vi "vision system.vi"() -> ()   [LabVIEW 2018]
uses:
  <vilib>/userdefined/High Color/IMAQdx.ctl
  <vilib>/vision/Measure.llb/Straight Edge Options.ctl
  <vilib>/vision/Measure.llb/Straight Edge Process.ctl
  <vilib>/vision/Measure.llb/Edge Options.ctl
  <vilib>/vision/Measure.llb/Edge Polarity.ctl
  <vilib>/Utility/file.llb/Read Delimited Spreadsheet (string).vi
  <vilib>/Utility/file.llb/Read Delimited Spreadsheet (DBL).vi
  <vilib>/Utility/file.llb/Write Delimited Spreadsheet (DBL).vi
  <vilib>/vision/driver/NI_Vision_Acquisition_Software.lvlib
  <vilib>/vision/NI_Vision_Development_Module.lvlib
panel:
  out "Jednostka ostatnia":string
  out "Ostatnia zapisana wartość:":dbl
  in  "Zmiana zakresu":i32 min=0
  out "Miernik":string
  in  "Zmiana mierzonej wielkości":i32 min=0
  out "Zakresy w kolumnach":dbl[][](array[numeric])
  out "Naglowki":string[][](array[string])
  in  "Plik z zakresami":path=path "C:/Users/Darek/Desktop/mierniki_zakresy.csv"
  in  "Skoroszyt csv do zapisu pomiarów":path=path "C:/Users/Darek/Desktop/wyniki_pomiarow.csv"
  in  "Zapis":bool
  out "Mnożnik zakresu":dbl
  in  "Kierunek ruchu wskazówki":T1(ring)
  out "Jednostka kopia":string
  out "Kąt wskazówki":dbl
  in  "Tryb zoptymalizowany":bool=TRUE
  in  "Opcje linii wskazówki":T2={"Edge Polarity"=0, "Kernel Size"=3, "Width"=3, "Minimum Edge Strength"=10.0, "Interpolation Type"=enum."Bilinear Fixed", "Data Processing Method"=enum."Average"} {"Edge Polarity" items=["All Edges", "Rising Edges", "Falling Edges"]; "Minimum Edge Strength" format="%.2f"; "Width" step=2; "Kernel Size" step=2}
  in  "Kierunek szukania":u32(ring) items=["Left to Right", "Right to Left", "Top to Bottom", "Bottom to Top"]
  in  "Dopasownie linii wskazówki":T4={"Number of Lines"=1, "Type"=enum."Best Edge Rake", "Min. Score"=10.0, "Max. Score"=1000.0, "Orientation"=0.0, "Angle Range"=10.0, "Angle Tolerance"=1.0, "Step Size"=3, "Min. SNR (db)"=0.0, "Min. Points (%)"=25.0, "Hough Iterations"=5} {"Min. Points (%)" min=0.0 max=100.0; "Min. SNR (db)" min=0.0; "Max. Score" min=0.0 max=1024.0; "Min. Score" min=0.0 max=1024.0 step=1.0}
  out "Kąt prawej linii":dbl
  out "Kąt lewej linii":dbl
  out "WYNIK":dbl
  out "Jednostka":string
  out "Zakres":dbl
  in  "Rodzaj skali":enum16{"Skale liniowe", "Ohmy V640"}(ring)
  in  "Znajdowanie \nwskazówki":bool
  out "Boolean 3":bool
  out "Kąt wskazówki raw":dbl
  out "Rozstaw podziałki\n w stopniach":dbl
  out "Kąt prawej linii raw":dbl
  out "Kąt lewej linii raw":dbl
  in  "Opcje prawej linii":T6={"Search Direction"=1, "Edge Options"={"Edge Polarity"=1, "Kernel Size"=3, "Width"=3, "Minimum Edge Strength"=10.0, "Interpolation Type"=enum."Bilinear Fixed", "Data Processing Method"=enum."Average"}, "Show Search Area"=FALSE, "Show Search Lines"=FALSE, "Show Edges Found"=FALSE, "Show Result"=FALSE, "Search Area Color"=65280, "Search Lines Color"=255, "Edge Locations Color"=16776960, "Result Color"=16711680, "Overlay Group Name"=""} {"Edge Options"."Edge Polarity" items=["All Edges", "Rising Edges", "Falling Edges"]; "Edge Options"."Minimum Edge Strength" format="%.2f"; "Edge Options"."Width" step=2; "Edge Options"."Kernel Size" step=2; "Search Direction" items=["Left to Right", "Right to Left", "Top to Bottom", "Bottom to Top"]}
  in  "Opcje lewej linii":T6={"Search Direction"=0, "Edge Options"={"Edge Polarity"=1, "Kernel Size"=3, "Width"=3, "Minimum Edge Strength"=10.0, "Interpolation Type"=enum."Bilinear Fixed", "Data Processing Method"=enum."Average"}, "Show Search Area"=FALSE, "Show Search Lines"=FALSE, "Show Edges Found"=FALSE, "Show Result"=FALSE, "Search Area Color"=65280, "Search Lines Color"=255, "Edge Locations Color"=16776960, "Result Color"=16711680, "Overlay Group Name"=""} {"Edge Options"."Edge Polarity" items=["All Edges", "Rising Edges", "Falling Edges"]; "Edge Options"."Minimum Edge Strength" format="%.2f"; "Edge Options"."Width" step=2; "Edge Options"."Kernel Size" step=2; "Search Direction" items=["Left to Right", "Right to Left", "Top to Bottom", "Bottom to Top"]}
  in  "Dop. prawej linii":T4={"Number of Lines"=1, "Type"=enum."First Edge Rake", "Min. Score"=10.0, "Max. Score"=1000.0, "Orientation"=0.0, "Angle Range"=45.0, "Angle Tolerance"=1.0, "Step Size"=7, "Min. SNR (db)"=0.0, "Min. Points (%)"=25.0, "Hough Iterations"=5} {"Min. Points (%)" min=0.0 max=100.0; "Min. SNR (db)" min=0.0; "Max. Score" min=0.0 max=1024.0; "Min. Score" min=0.0 max=1024.0 step=1.0}
  out "Boolean 2":bool
  in  "Znajdowanie \nprostych":bool
  out "Boolean":bool
  in  "Dopasowanie \nwzorca":bool
  in  "Dop. lewej linii":T4={"Number of Lines"=1, "Type"=enum."First Edge Rake", "Min. Score"=10.0, "Max. Score"=1000.0, "Orientation"=0.0, "Angle Range"=45.0, "Angle Tolerance"=1.0, "Step Size"=7, "Min. SNR (db)"=0.0, "Min. Points (%)"=25.0, "Hough Iterations"=5} {"Min. Points (%)" min=0.0 max=100.0; "Min. SNR (db)" min=0.0; "Max. Score" min=0.0 max=1024.0; "Min. Score" min=0.0 max=1024.0 step=1.0}
  out "Podglad":T7(plugin-control)
  out "Miernik wykryty":bool
  in  "stop":bool
  out "Błąd pracy systemu":errorcluster
  out "Wzorzec":T7(plugin-control)
  in  "Paramtery\ndopasowania":T8={"Number of Matches Requested"=1, "Minimum Match Score"=800.0, "Angle Ranges"=[]}
  in  "Sciezka \nobrazu wzorcowego":path=path "C:/Users/Darek/Desktop/templates/V640_temp_8bit.png"
  out "Błąd akwizycji obrazu":errorcluster
  in  "Kamera":T9="cam1"
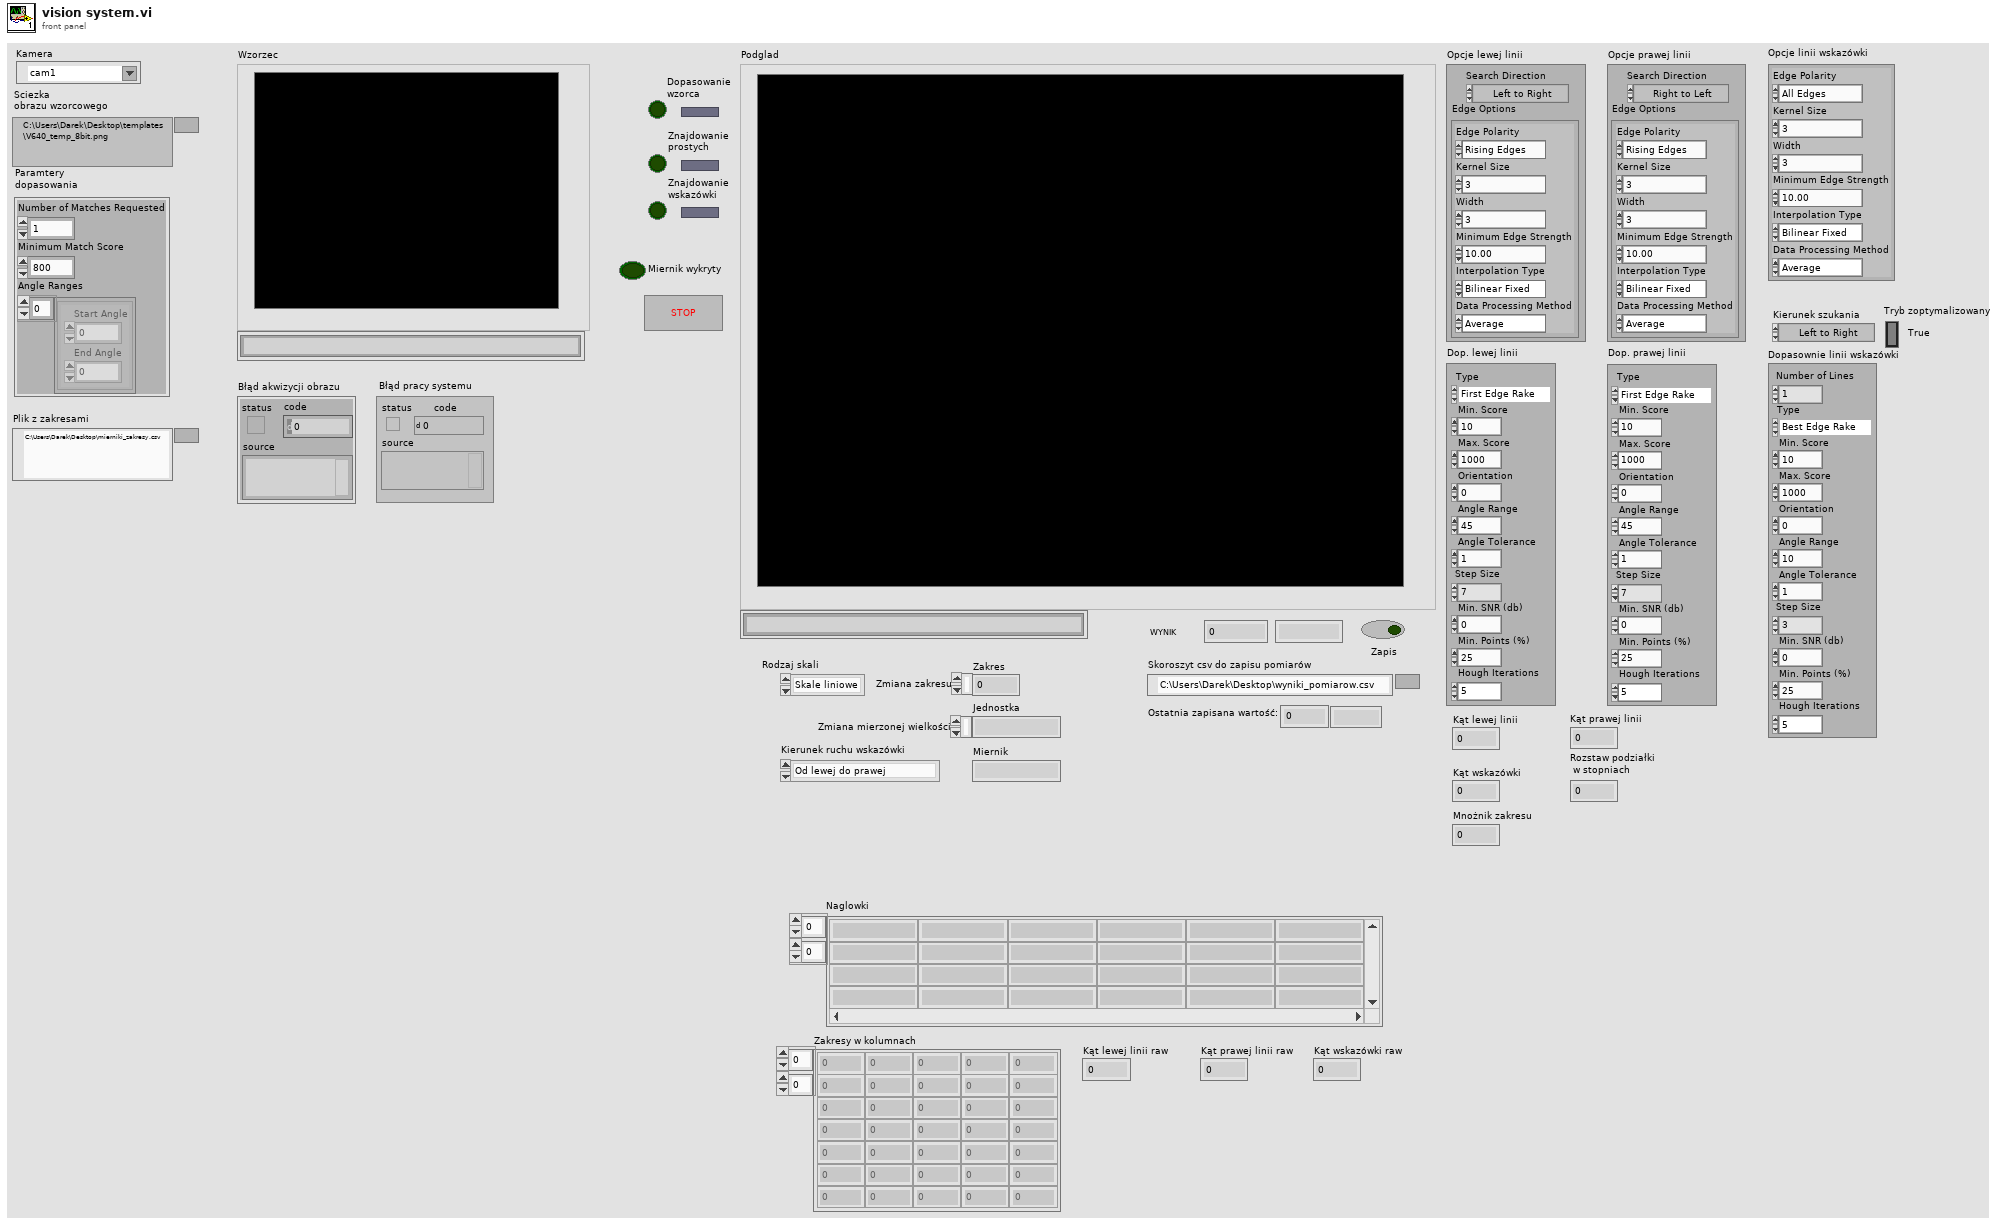
[diagram p1: front panel]
types:
  T1 = enum16{"Od lewej do prawej", "Od prawej do lewej"}
  T2 = typedef "Edge Options.ctl" = cluster{"Edge Polarity":T3, "Kernel Size":u32, "Width":u32, "Minimum Edge Strength":sgl, "Interpolation Type":enum32{"Zero Order", "Bilinear", "Quadratic", "Cubic", "Bilinear Fixed"}, "Data Processing Method":enum32{"Average", "Median"}}
  T3 = typedef "Edge Polarity.ctl" = u32
  T4 = typedef "Straight Edge Options.ctl" = cluster{"Number of Lines":i32, "Type":T5, "Min. Score":dbl, "Max. Score":dbl, "Orientation":dbl, "Angle Range":dbl, "Angle Tolerance":dbl, "Step Size":u32, "Min. SNR (db)":dbl, "Min. Points (%)":dbl, "Hough Iterations":i32}
  T5 = typedef "Straight Edge Process.ctl" = enum32{"First Edge Rake", "Best Edge Rake", "Hough Edge Rake", "First Edge Projection", "Best Edge Projection"}
  T6 = cluster{"Search Direction":u32, "Edge Options":T2, "Show Search Area":bool, "Show Search Lines":bool, "Show Edges Found":bool, "Show Result":bool, "Search Area Color":u32, "Search Lines Color":u32, "Edge Locations Color":u32, "Result Color":u32, "Overlay Group Name":string}
  T7 = typedef "IMAQ Image.ctl" = refnum<image>
  T8 = cluster{"Number of Matches Requested":i32, "Minimum Match Score":sgl, "Angle Ranges":cluster{"Start Angle":sgl, "End Angle":sgl}[]}
  T9 = typedef "IMAQdx.ctl" = refnum<k21>
  T10 = typedef "Image Type" = u32
  T11 = cluster{i32, "Y Resolution":i32, "X Resolution":i32, i32, dbl}
  T12 = typedef "ROI Descriptor" = cluster{"Global Rectangle":i32[], "Contours":cluster{"ID":enum32{"External", "Internal"}, "Type":u32, "Coordinates":i32[]}[]}
  T13 = cluster{"Position":cluster{"x":sgl, "y":sgl}, "Angle":sgl, "Scale":sgl, "Score":sgl, "Bounding Box":cluster{"x":sgl, "y":sgl}[]}[]
  T14 = typedef "IMAQ Coordinate System" = cluster{"Reference System":cluster{"Origin":cluster{"X":sgl, "Y":sgl}, "Angle (deg)":sgl, "Axis Reference":u32}, "Measurement System":cluster{"Origin":cluster{"X":sgl, "Y":sgl}, "Angle (deg)":sgl, "Axis Reference":u32}}
  T15 = cluster{"Point1 (Pixels)":cluster{"X":sgl, "Y":sgl}, "Point2 (Pixels)":cluster{"X":sgl, "Y":sgl}, "Point1 (Real-World)":cluster{"X":sgl, "Y":sgl}, "Point2 (Real-World)":cluster{"X":sgl, "Y":sgl}, "Angle (Pixel)":dbl, "Angle (Real-World)":dbl, "Score":dbl, "Straightness":dbl, "Average SNR (db)":dbl, "Calibration Valid":bool}[]
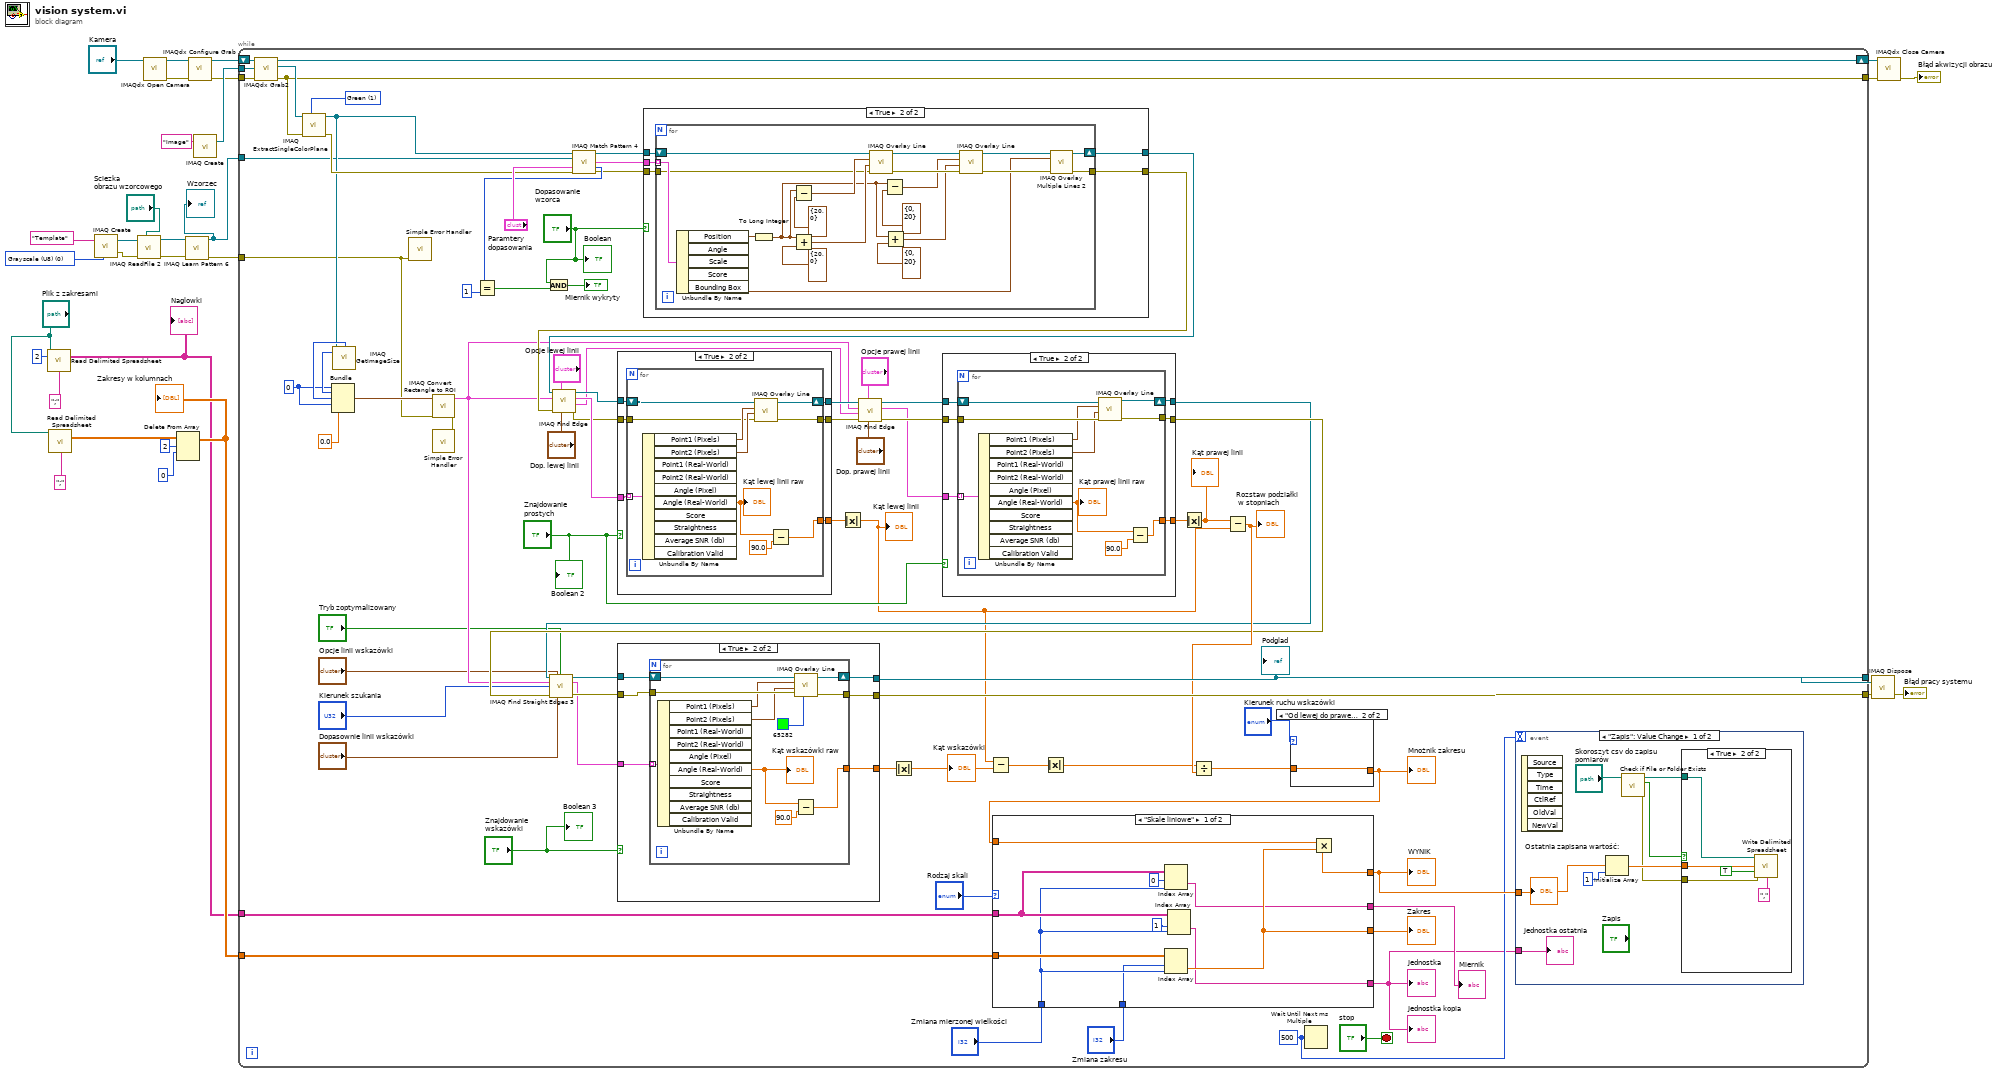
[diagram p0: block diagram]
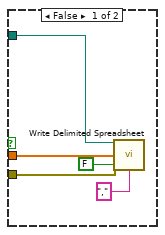
[diagram p2: hidden frame]
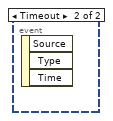
[diagram p3: hidden frame]
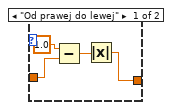
[diagram p4: hidden frame]
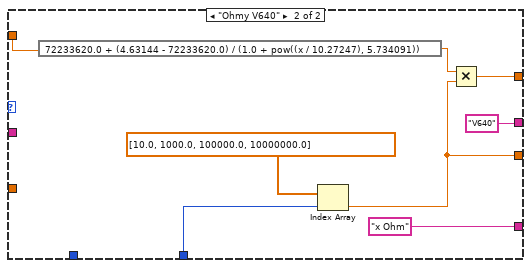
[diagram p5: hidden frame]
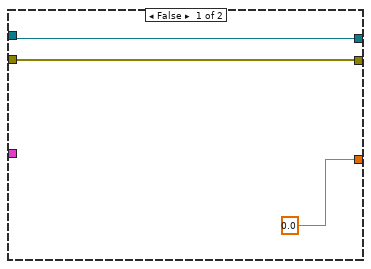
[diagram p6: hidden frame]
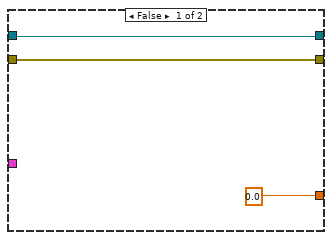
[diagram p7: hidden frame]
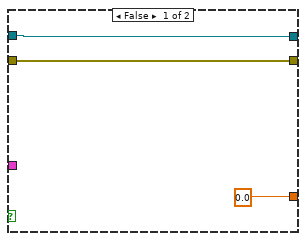
[diagram p8: hidden frame]
diagram:
  w19 = T10 0 items=["Grayscale (U8)", "Grayscale (I16)", "Grayscale (SGL)", "Complex (CSG)", "RGB (U32)", "HSL (U32)", "RGB (U64)", "Grayscale (U16)"] ("Image Type")
  n1 = call-poly <vilib>:"Read Delimited Spreadsheet.vi"("file path (dialog if empty)"="Plik z zakresami", "number of rows (all:-1)"=2, "delimiter (\\t)"=";" ("delimiter (\\t)")) -> ("all rows"=w1:string[][])  [unwired: 7 in, 5 out]
  "Naglowki" <- w1
  n2 = call-poly <vilib>:"Read Delimited Spreadsheet.vi"("file path (dialog if empty)"="Plik z zakresami", "delimiter (\\t)"=";" ("delimiter (\\t)")) -> ("all rows"=w5:dbl[][])  [unwired: 8 in, 5 out]
  n3 = call "IMAQ Create"("Image Name"="Template", "Image Type"=w19) -> ("New Image"=w15:T7, "error out"=w16:errorcluster)  [unwired: 3 in]
  n4 = call "IMAQ ReadFile 2"("File Path"="Sciezka \nobrazu wzorcowego", "error in (no error)"=w16, "Image"=w15) -> ("error out"=w14:errorcluster, "Image Out"=w12:T7)  [unwired: 4 in, 3 out]
  n5 = call <vilib>:"IMAQdx Open Camera.vi"("Session In"="Kamera") -> ("error out"=w28:errorcluster, "Session Out"=w31:T9)  [unwired: 9 in]
  n6 = Delete From Array(array=w5, length=2, index (row)=0) -> (array with subset deleted=w2:dbl[][])  [unwired: 1 in, 1 out]
  "Zakresy w kolumnach" <- w2
  n7 = call "IMAQ Learn Pattern 6"("Image"=w12, "error in (no error)"=w14) -> ("Template Image Out"=w11:T7, "error out"=w10:errorcluster)  [unwired: 11 in, 1 out]
  "Wzorzec" <- w11
  n8 = call <vilib>:"IMAQdx Configure Grab.vi"("error in"=w28, "Session In"=w31) -> ("error out"=w22:errorcluster, "Session Out"=w30:T9)  [unwired: 8 in]
  n9 = call "IMAQ Create"("Image Name"="Image") -> ("New Image"=w24:T7)  [unwired: 4 in, 1 out]
  n10 = while {
    shift-right: [w108] -> w27
    shift-left: w30 -> [w109]
    tunnel: w24 -> [w105]
    tunnel: w22 -> [w101]
    tunnel: [w100] -> w21
    tunnel: [w70] -> w18
    tunnel: [w67] -> w17
    tunnel: w11 -> [w39]
    tunnel: w10 -> [w38]
    tunnel: w2 -> [w37]
    tunnel: w1 -> [w36]
    stop <- "stop" stop-if-true
    w40 = u32 500 ("millisecond multiple")
    w89 = 0
    w106 = 1 items=["Red", "Green", "Blue", "Hue", "Saturation", "Luminance", "Value", "Intensity"] ("Color Plane")
    n11 = call <vilib>:"IMAQdx Grab2.vi"("error in"=w101, "Image In"=w105, "Session In"=w109) -> ("error out"=w100:errorcluster, "Image Out"=w107:T7, "Session Out"=w108:T9)  [unwired: 5 in, 1 out]
    n12 = call "IMAQ ExtractSingleColorPlane"("Color Plane"=w106, "error in (no error)"=w100, "Image Src"=w107) -> ("error out"=w94:errorcluster, "Image Dst Out"=w86:T7)  [unwired: 7 in]
    n13 = call "IMAQ GetImageSize"("Image"=w86) -> ("Y Resolution"=w91:i32, "X Resolution"=w90:i32)  [unwired: 3 in, 1 out]
    n14 = Bundle(w89, "Y Resolution"=w91, "X Resolution"=w90, w89, 0.0) -> (w87:T11)  [unwired: 1 in]
    n15 = call <vilib>:"Simple Error Handler.vi"("error in (no error)"=w38) -> ()  [unwired: 4 in, 5 out]
    n16 = call "IMAQ Convert Rectangle to ROI"("error in (no error)"=w38, "Rectangle"=w87) -> ("error out"=w92:errorcluster, "ROI Descriptor"=w54:T12)  [unwired: 7 in]
    n17 = call <vilib>:"Simple Error Handler.vi"("error in (no error)"=w92) -> ()  [unwired: 4 in, 5 out]
    n18 = call "IMAQ Match Pattern 4"("Image"=w86, "Template Image"=w39, "Parameters"="Paramtery\ndopasowania", "error in (no error)"=w94) -> ("Image (duplicate)"=w64:T7, "Matches (pixel)"=w63:T13, "Number of Matches"=w62:i32, "error out"=w61:errorcluster)  [unwired: 7 in, 1 out]
    n19 = Equal?(x=w62, y=1) -> (x = y?=w85:bool)
    n20 = And(x="Dopasowanie \nwzorca", y=w85) -> (x .and. y?=→"Miernik wykryty":bool)
    n21 = case shown="True" "Dopasowanie \nwzorca" {
      tunnel: w64 -> [w211 w216]
      tunnel: w61 -> [w210 w215]
      tunnel: w63 -> [_ w214]
      tunnel: [w211 w213] -> w95
      tunnel: [w210 w212] -> w93
      frame False {
      }
      frame True {
        n22 = for {
          shift-right: [w217] -> w213
          shift-left: w216 -> [w221]
          tunnel: w214 -> [w232] mode=indexing
          tunnel: w215 -> [w220]
          tunnel: [w219] -> w212
          n23 = Unbundle By Name(w232) -> ("Position"=w231:cluster{"x":sgl, "y":sgl}, "Bounding Box"=w218:cluster{"x":sgl, "y":sgl}[])  [unwired: 3 out]
          n24 = To Long Integer(number=w231) -> (32bit integer=w225:cluster{"x":i32, "y":i32})
          n25 = Subtract(x=w225, y=cluster{"x":i32, "y":i32} {"x"=20, "y"=0}) -> (x-y=w228:cluster{"x":i32, "y":i32})
          n26 = Add(x=w225, y=cluster{"x":i32, "y":i32} {"x"=20, "y"=0}) -> (x+y=w227:cluster{"x":i32, "y":i32})
          n27 = call "IMAQ Overlay Line"("error in (no error)"=w220, "End Point"=w227, "Start Point"=w228, "Image"=w221) -> ("error out"=w234:errorcluster, "Image Out"=w235:T7)  [unwired: 6 in]
          n28 = Subtract(x=w225, y=cluster{"x":i32, "y":i32} {"x"=0, "y"=20}) -> (x-y=w223:cluster{"x":i32, "y":i32})
          n29 = Add(x=w225, y=cluster{"x":i32, "y":i32} {"x"=0, "y"=20}) -> (x+y=w222:cluster{"x":i32, "y":i32})
          n30 = call "IMAQ Overlay Line"("error in (no error)"=w234, "End Point"=w222, "Start Point"=w223, "Image"=w235) -> ("error out"=w236:errorcluster, "Image Out"=w233:T7)  [unwired: 6 in]
          n31 = call "IMAQ Overlay Multiple Lines 2"("Image"=w233, "Line End Points"=w218, "error in (no error)"=w236) -> ("Image Out"=w217:T7, "error out"=w219:errorcluster)  [unwired: 11 in]
        }
      }
    }
    n32 = call "IMAQ Find Edge"("Line Fit Options"="Dop. lewej linii", "Options"="Opcje lewej linii", "error in (no error)"=w93, "ROI Descriptor"=w54, "Image"=w95) -> ("error out"=w96:errorcluster, "Coordinate System (duplicate)"=w74:T14, "Straight Edges"=w98:T15, "Image Out"=w97:T7)  [unwired: 3 in]
    n33 = case shown="True" "Znajdowanie \nprostych" {
      tunnel: w98 -> [_ w199]
      tunnel: w97 -> [w193 w198]
      tunnel: [w193 w197] -> w83
      tunnel: w96 -> [w192 w196]
      tunnel: [w192 w195] -> w82
      tunnel: [0.0 w194] -> w73
      frame False {
      }
      frame True {
        n34 = for {
          tunnel: w199 -> [w209] mode=indexing
          shift-right: [w207] -> w197
          shift-left: w198 -> [w208]
          tunnel: w196 -> [w204]
          tunnel: [w203] -> w195
          tunnel: [w200] -> w194
          n35 = Unbundle By Name(w209) -> ("Point1 (Pixels)"=w206:cluster{"X":sgl, "Y":sgl}, "Point2 (Pixels)"=w205:cluster{"X":sgl, "Y":sgl}, "Angle (Real-World)"=w202:dbl)  [unwired: 7 out]
          "Kąt lewej linii raw" <- w202
          n36 = call "IMAQ Overlay Line"("error in (no error)"=w204, "End Point"=w205, "Start Point"=w206, "Image"=w208) -> ("error out"=w203:errorcluster, "Image Out"=w207:T7)  [unwired: 6 in]
          n37 = Subtract(x=w202, y=90.0) -> (x-y=w200:dbl)
        }
      }
    }
    n38 = Absolute Value(x=w73) -> (abs(x)=w48:dbl)
    "Kąt lewej linii" <- w48
    n39 = call "IMAQ Find Edge"("Line Fit Options"="Dop. prawej linii", "Options"="Opcje prawej linii", "error in (no error)"=w82, "Coordinate System"=w74, "ROI Descriptor"=w54, "Image"=w83) -> ("error out"=w79:errorcluster, "Straight Edges"=w78:T15, "Image Out"=w80:T7)  [unwired: 2 in, 1 out]
    n40 = case shown="True" "Znajdowanie \nprostych" {
      tunnel: [w174 w177] -> w56
      tunnel: w80 -> [w174 w178]
      tunnel: [w173 w179] -> w57
      tunnel: w79 -> [w173 w180]
      tunnel: w78 -> [_ w176]
      tunnel: [0.0 w175] -> w72
      frame False {
      }
      frame True {
        n41 = for {
          tunnel: w180 -> [w190]
          tunnel: [w189] -> w179
          shift-right: [w187] -> w177
          shift-left: w178 -> [w188]
          tunnel: w176 -> [w186] mode=indexing
          tunnel: [w181] -> w175
          n42 = Unbundle By Name(w186) -> ("Point1 (Pixels)"=w185:cluster{"X":sgl, "Y":sgl}, "Point2 (Pixels)"=w184:cluster{"X":sgl, "Y":sgl}, "Angle (Real-World)"=w183:dbl)  [unwired: 7 out]
          "Kąt prawej linii raw" <- w183
          n43 = call "IMAQ Overlay Line"("error in (no error)"=w190, "End Point"=w184, "Start Point"=w185, "Image"=w188) -> ("error out"=w189:errorcluster, "Image Out"=w187:T7)  [unwired: 6 in]
          n44 = Subtract(x=w183, y=90.0) -> (x-y=w181:dbl)
        }
      }
    }
    n45 = call "IMAQ Find Straight Edges 3"("Image"=w56, "Edge Options"="Opcje linii wskazówki", "Optimized Mode"="Tryb zoptymalizowany", "ROI Descriptor"=w54, "Search Direction"="Kierunek szukania", "error in (no error)"=w57, "Line Options"="Dopasownie linii wskazówki") -> ("Image (duplicate)"=w55:T7, "Straight Edges"=w49:T15, "error out"=w58:errorcluster)  [unwired: 4 in, 2 out]
    n46 = case shown="True" "Znajdowanie \nwskazówki" {
      tunnel: w58 -> [w154 w160]
      tunnel: [w154 w159] -> w70
      tunnel: [w152 w158] -> w67
      tunnel: [0.0 w155] -> w68
      tunnel: w55 -> [w152 w157]
      tunnel: w49 -> [_ w156]
      frame False {
      }
      frame True {
        n47 = for {
          tunnel: w160 -> [w171]
          tunnel: [w170] -> w159
          shift-right: [w168] -> w158
          shift-left: w157 -> [w169]
          tunnel: w156 -> [w166] mode=indexing
          tunnel: [w161] -> w155
          n48 = Unbundle By Name(w166) -> ("Point1 (Pixels)"=w165:cluster{"X":sgl, "Y":sgl}, "Point2 (Pixels)"=w164:cluster{"X":sgl, "Y":sgl}, "Angle (Real-World)"=w162:dbl)  [unwired: 7 out]
          "Kąt wskazówki raw" <- w162
          n49 = call "IMAQ Overlay Line"("Color"=u32 65282, "error in (no error)"=w171, "End Point"=w164, "Start Point"=w165, "Image"=w169) -> ("error out"=w170:errorcluster, "Image Out"=w168:T7)  [unwired: 5 in]
          n50 = Subtract(x=w162, y=90.0) -> (x-y=w161:dbl)
        }
      }
    }
    "Podglad" <- w67
    n51 = Absolute Value(x=w68) -> (abs(x)=w47:dbl)
    "Kąt wskazówki" <- w47
    n52 = Subtract(x=w48, y=w47) -> (x-y=w46:dbl)
    n53 = Absolute Value(x=w46) -> (abs(x)=w45:dbl)
    n54 = Absolute Value(x=w72) -> (abs(x)=w71:dbl)
    "Kąt prawej linii" <- w71
    n55 = Subtract(x=w71, y=w48) -> (x-y=w66:dbl)
    "Rozstaw podziałki\n w stopniach" <- w66
    n56 = Divide(x=w45, y=w66) -> (x/y=w43:dbl)
    n57 = case shown="\"Od lewej do prawej\", Default" "Kierunek ruchu wskazówki" {
      tunnel: [w128 w132] -> w42
      tunnel: w43 -> [w131 w132]
      frame "Od prawej do lewej" {
        n58 = Subtract(x=1.0, y=w131) -> (x-y=w129:dbl)
        n59 = Absolute Value(x=w129) -> (abs(x)=w128:dbl)
      }
      frame "Od lewej do prawej", Default {
      }
    }
    "Mnożnik zakresu" <- w42
    n60 = case shown="\"Skale liniowe\"" "Rodzaj skali" {
      tunnel: [w142 w147] -> w59
      tunnel: [w138 "x Ohm"] -> w32
      tunnel: w42 -> [w143 w149]
      tunnel: [w141 w146] -> w41
      tunnel: w37 -> [w140 _]
      tunnel: w36 -> [w139 _]
      tunnel: "Zmiana mierzonej wielkości" -> [w134 _]
      tunnel: [w137 "V640"] -> w34
      tunnel: "Zmiana zakresu" -> [w133 w144]
      frame "Skale liniowe" {
        n61 = Index Array(array=w139, index (row)=0 ("disabled index (row)"), index (col)=w134) -> (element=w137:string)
        n62 = Index Array(array=w140, index (row)=w133, index (col)=w134) -> (element=w142:dbl)
        n63 = Index Array(array=w139, index (row)=1, index (col)=w134) -> (element=w138:string)
        n64 = Multiply(x=w143, y=w142) -> (x*y=w141:dbl)
      }
      frame "Ohmy V640" {
        n65 = expression code="72233620.0 + (4.63144 - 72233620.0) / (1.0 + pow((x / 10.27247), 5.734091))"(w149) -> (w148:dbl)
        n66 = Index Array(array=dbl[] [10.0, 1000.0, 100000.0, 10000000.0], index=w144) -> (element=w147:dbl)
        n67 = Multiply(x=w148, y=w147) -> (x*y=w146:dbl)
      }
    }
    "Zakres" <- w59
    "Jednostka" <- w32
    "WYNIK" <- w41
    "Jednostka kopia" <- w32
    "Miernik" <- w34
    n68 = Wait Until Next ms Multiple(millisecond multiple=w40) -> ()  [unwired: 1 out]
    n69 = event shown="[0] \"Zapis\": Value Change" {
      selector: _ -> [_ _]
      dyn-events: _ -> [_ _]
      timeout: w40 -> [_ _]
      tunnel: w41 -> [w111 _]
      tunnel: w32 -> [w110 _]
      event "Zapis": Value Change {
        n70 = event-data() -> ()  [unwired: 1 in, 6 out]
        n71 = Initialize Array(w111, 1 ("dimension size")) -> (w114:dbl[])
        n72 = call <vilib>:"Check if File or Folder Exists.vi"("path"="Skoroszyt csv do zapisu pomiarów") -> ("error out"=w113:errorcluster, "file or folder exists?"=w116:bool, "dup path"=w115:path)  [unwired: 8 in]
        n73 = case shown="True" w116 {
          tunnel: w115 -> [w120 w127]
          tunnel: w114 -> [w119 w126]
          tunnel: w113 -> [w118 w125]
          frame False {
            n74 = call-poly <vilib>:"Write Delimited Spreadsheet.vi"("file path (dialog if empty)"=w120, "1D data"=w119, "append to file? (new file:F)"=FALSE, "error in (no error)"=w118, "delimiter (\\t)"="," ("delimiter (\\t)")) -> ()  [unwired: 9 in, 2 out]
          }
          frame True {
            n75 = call-poly <vilib>:"Write Delimited Spreadsheet.vi"("file path (dialog if empty)"=w127, "1D data"=w126, "append to file? (new file:F)"=TRUE, "error in (no error)"=w125, "delimiter (\\t)"="," ("delimiter (\\t)")) -> ()  [unwired: 9 in, 2 out]
          }
        }
        "Ostatnia zapisana wartość:" <- w111
        "Jednostka ostatnia" <- w110
      }
      event Timeout {
        n76 = event-data() -> ()  [unwired: 1 in, 3 out]
      }
    }
    "Boolean" <- "Dopasowanie \nwzorca"
    "Boolean 2" <- "Znajdowanie \nprostych"
    "Boolean 3" <- "Znajdowanie \nwskazówki"
  }
  n77 = call "IMAQ Dispose"("Image"=w17, "error in (no error)"=w18) -> ("error out"=→"Błąd pracy systemu":errorcluster)  [unwired: 4 in]
  n78 = call <vilib>:"IMAQdx Close Camera.vi"("error in"=w21, "Session In"=w27) -> ("error out"=→"Błąd akwizycji obrazu":errorcluster)  [unwired: 9 in]
